vi "Build Path Model.vi"(8 "error in":errorcluster, 11 "Report Generator in":refnum<class "Report Generator.lvclass">) -> (0 "error out":errorcluster, 3 "Report Generator out":refnum<class "Report Generator.lvclass">)   [LabVIEW 2018, in "Report Generator.lvlib" / "Report Generator.lvclass"]
uses:
  Report Generator.lvclass
  Report Generator.lvclass/Report Generator.ctl
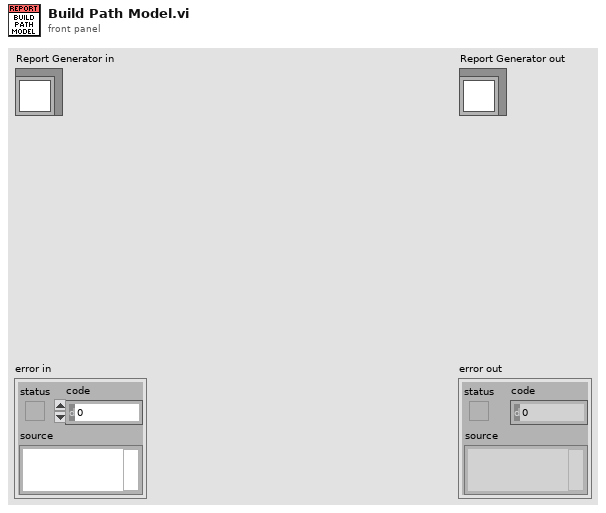
[diagram p1: front panel]
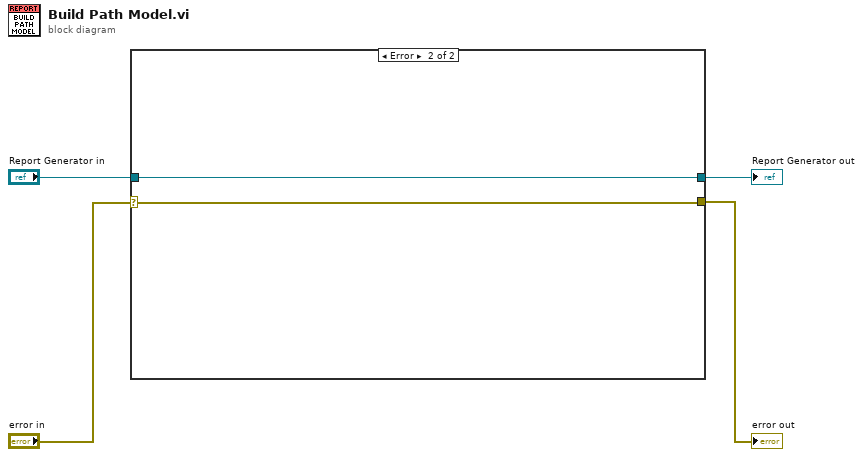
[diagram p0: block diagram]
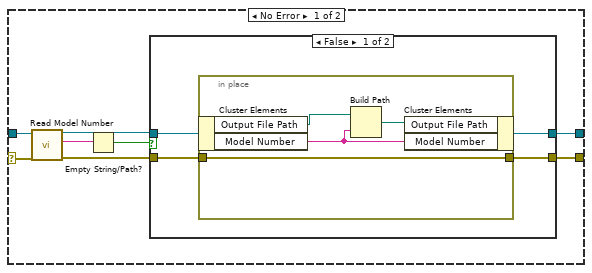
[diagram p2: hidden frame]
diagram:
  n1 = case shown="Error" "error in" {
    selector: "error in" -> [w6 w23]
    tunnel: "Report Generator in" -> [w12 w24]
    tunnel: [w7 w24] -> w3
    tunnel: [w5 w23] -> w1
    frame No Error {
      n2 = call "Read Model Number.vi"("error in (no error)"=w6, "Report Generator in"=w12) -> ("error out"=w8:errorcluster, "Model Number"=w11:string, "Report Generator out"=w9:refnum<class "Report Generator.lvclass">)  [unwired: 7 in]
      n3 = Empty String/Path?(string/path=w11) -> (empty?=w10:bool)
      n4 = case shown="False" w10 {
        tunnel: w9 -> [w16 w21]
        tunnel: w8 -> [w14 w22]
        tunnel: [w13 w22] -> w5
        tunnel: [w15 w21] -> w7
        frame False {
          n5 = in-place {
            in-place-border: w14 -> [w20]
            in-place-border: [w20] -> w13
            n6 = in-place-cluster #1(w16) -> ("Output File Path"=w19:path, "Model Number"=w18:string)
            n7 = Build Path(base path=w19, name or relative path=w18) -> (appended path=w17:path)
            n8 = in-place-cluster #1("Output File Path"=w17, "Model Number"=w18) -> (w15:refnum<class "Report Generator.lvclass">)
          }
        }
        frame True {
        }
      }
    }
    frame Error {
    }
  }
  "error out" <- w1
  "Report Generator out" <- w3
